vi "PODYEZD.vi"   [LabVIEW 2018]
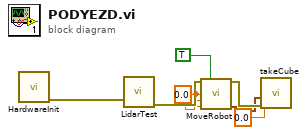
[diagram p0: block diagram]
diagram:
  w4 = 0.0 ("x (mm/s)")
  n1 = call "HardwareInit.vi"() -> ("error out"=w7:errorcluster)  [unwired: 11 in]
  n2 = call "LidarTest.vi"("Error/Flow In"=w7) -> ("Error/Flow Out"=w5:errorcluster)  [unwired: 10 in]
  n3 = call "MoveRobot.vi"("Error/Flow In"=w5, "Reset"=TRUE, "x (mm/s)"=w4, "y (mm/s)"=w4, "theta (rad/s)"=w4) -> ("Error/Flow Out"=w3:errorcluster, "Position"=w2:cluster{"X":dbl, "Y":dbl, "Theta":dbl})  [unwired: 9 in]
  n4 = call "takeCube.vi"("Error/Flow In"=w3, "Position (mm)"=w2, "theta"=0.0) -> ()  [unwired: 7 in, 2 out]
